vi "Write Class Type.vi"(8 "error in (no error)":errorcluster, 10 "RHS class type":T1 items=["RHS"=0, "RHS_2D"=20, "RHS_2D_Numeric"=21, "RHS_2D_VIRef"=22, "RHS_3D"=30, "RHS_3D_Numeric"=31, "RHS_3D_VIRef"=32], 11 "RHS.lvclass in":refnum<class "NI_RHS.lvclass">) -> (0 "error out":errorcluster, 3 "RHS.lvclass out":refnum<class "NI_RHS.lvclass">)   [LabVIEW 2020, in "NI_PDE.lvlib" / "NI_RHS.lvclass"]
uses:
  <vilib>/gmath/pde.llb/RHSClass/NI_RHS.lvclass
  <vilib>/gmath/pde.llb/RHSClass/Class Type.ctl
  <vilib>/gmath/pde.llb/RHSClass/NI_RHS.lvclass/NI_RHS.ctl
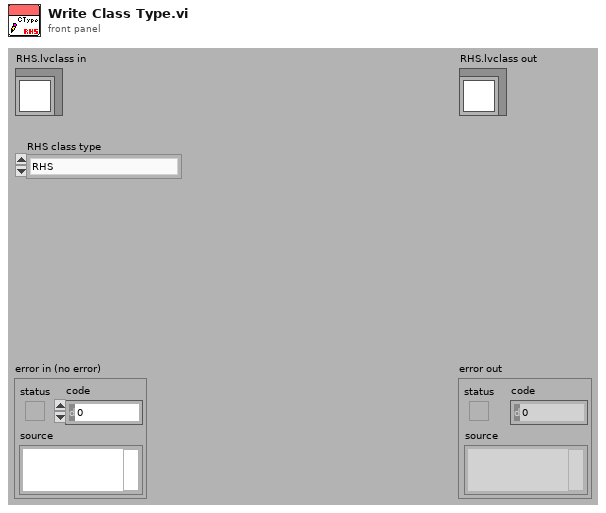
[diagram p1: front panel]
types:
  T1 = typedef "NI_PDE.lvlib/NI_RHS.lvclass/Class Type.ctl" = i32
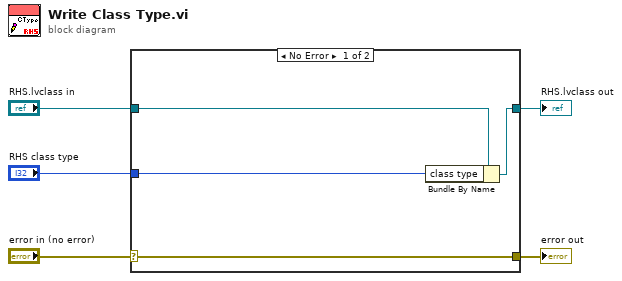
[diagram p0: block diagram]
diagram:
  n1 = case shown="No Error" "error in (no error)" {
    selector: "error in (no error)" -> [w9 w10]
    tunnel: [w9 w10] -> w4
    tunnel: [w7 w11] -> w2
    tunnel: "RHS.lvclass in" -> [w8 w11]
    tunnel: "RHS class type" -> [w6 _]
    frame No Error {
      n2 = Bundle By Name(cluster=w8, "class type"=w6) -> (w7:refnum<class "NI_RHS.lvclass">)
    }
    frame Error {
    }
  }
  "error out" <- w4
  "RHS.lvclass out" <- w2
